vi "Format Log to String.vi"(10 "Log Packet":T1, 11 "IStringFormat in":refnum<class "IStringFormat.lvclass">) -> (2 "Log Entry":string, 3 "IStringFormat out":refnum<class "IStringFormat.lvclass">)   [LabVIEW 2019, in "IStringFormat.lvclass"]
uses:
  <vilib>/gpm_packages/@cs/event-logger/Source/IStringFormat/IStringFormat.lvclass
  <vilib>/gpm_packages/@cs/event-logger/Source/Composed Log/Types/Log Packet.ctl
  <vilib>/gpm_packages/@cs/event-logger/Source/Composed Log/Types/Log Level.ctl
  <vilib>/gpm_packages/@cs/event-logger/Source/Composed Log/Composed Log.lvlib
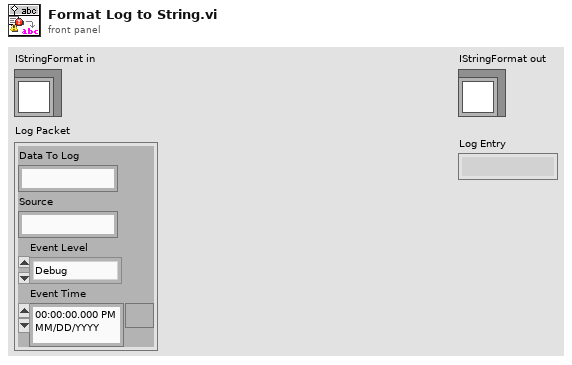
[diagram p1: front panel]
types:
  T1 = typedef "Composed Log.lvlib/Log Packet.ctl" = cluster{"Data To Log":string, "Source":string, "Event Level":T2, "Event Time":timestamp}
  T2 = typedef "Composed Log.lvlib/Log Level.ctl" = enum16{"Debug", "Info", "Warning", "Error", "Critical"}
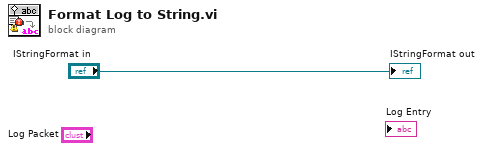
[diagram p0: block diagram]
diagram:
  "IStringFormat out" <- "IStringFormat in"
